vi "TDC Data Monitor def.9.vi"() -> ()   [LabVIEW 2011]
panel:
  out "Numeric 2":u32
  in  "Buffer size 2":u32=548
  out "Numeric":i32
  in  "stop 2":bool
  out "Active \nTimeout":bool
  in  "Buffer size":u32=548
  in  "Change UDP Parameters":bool
  out "Event Hex":string
  in  "see table channel  2":bool
  in  "see supertime sec":bool
  in  "see supertime  ns":bool
  in  "see channel":bool
  in  "see tot":bool
  in  "see table channel":bool
  out "error tdc not foud":bool
  out "Num Pack 2":u32=1
  out "Supertime ns":u32=1
  out "Supertime sec":u32=1
  out "error time order":bool
  out "error channel":bool
  out "Num Pack":u32=1
  out "Veces canal":u32[](array[numeric])
  out "Table":string[][](table)
  out "num canal":i32=548
  out "Canal TDC":u32[](array[numeric])
  in  "desviacion tipica ancho":dbl
  in  "suma desviacon":dbl
  out "media pulso":dbl
  in  "suma ancho pulso":u32=1
  out "iteracion":i32
  in  "stop":bool
  out "error timestamp":bool
  out "TOT":dynamicdata(graph) caption="Histogram"
  out "CHANNEL":dynamicdata(graph) caption="Histogram"
  out "ToT":u32=1
  out "Arrival Time":u32=1
  out "Channel TDC":u32=1
  out "bufferfull":timestamp
  out "UDP INDEX":dynamicdata(graph) caption="Histogram"
  out "EVENT/TS":dynamicdata(graph) caption="Histogram"
  out "indice":u32=1
  out "Supertime sec":dynamicdata(graph)
  out "supertime ns":dynamicdata(graph)
  out "current_HRV":u32=1
  out "current_fifo_afull":u32=1
  out "FIFO_FULL":bool[](array[boolean])
  out "HRV":bool[](array[boolean])
  out "Size Packet Bytes":i32
  out "Data Received":string
  out "Timeout UDP READ  ms":i32
  out "max bytes/read":i32=548
  in  "index":u32=1
  in  "Port":u16=61557
  out "Receive Buffer Size":u32
  out "Num Event":u32=1
  out "START TIME":timestamp
  out "hold_fifo_afull":u32=1
  out "hold_HRV":u32=1
  in  "event/ts":u32=1
  in  "pak_loss":u32=1 caption="packet losses"
  in  "TS_Ch_1":u32=1
  in  "TS_Ch 2":u32=1
  in  "TS_Ch 3":u32=1
  in  "TS_Ch 4":u32=1
  in  "TS_Ch 5":u32=1
  in  "TS_Ch 6":u32=1
  in  "TS_Ch 7":u32=1
  in  "TS_Ch 8":u32=1
  in  "TS_Ch 9":u32=1
  in  "TS_Ch 10":u32=1
  in  "TS_Ch_0":u32=1
  in  "TS_Ch_13":u32=1
  in  "TS_Ch 12":u32=1
  in  "TS_Ch_14":u32=1
  in  "TS_Ch_11":u32=1
  in  "TS_Ch_15":u32=1
  in  "TS_Ch_16":u32=1
  in  "TS_Ch_18":u32=1
  in  "TS_Ch 19":u32=1
  in  "TS_Ch_20":u32=1
  in  "TS_Ch_17":u32=1
  in  "TS_Ch_21":u32=1
  in  "TS_Ch_22":u32=1
  in  "TS_Ch_24":u32=1
  in  "TS_Ch 25":u32=1
  in  "TS_Ch_26":u32=1
  in  "TS_Ch_23":u32=1
  in  "TS_Ch_27":u32=1
  in  "TS_Ch_28":u32=1
  in  "TS_Ch_29":u32=1
  in  "TS_Ch_30":u32=1
  # "TDC DATA MONITOR"
  # "UDP TRANSFER CONDITIONS"
  # "PACKET INFORMATION"
  # "EVENT INFORMATION"
  # "See table of channel events"
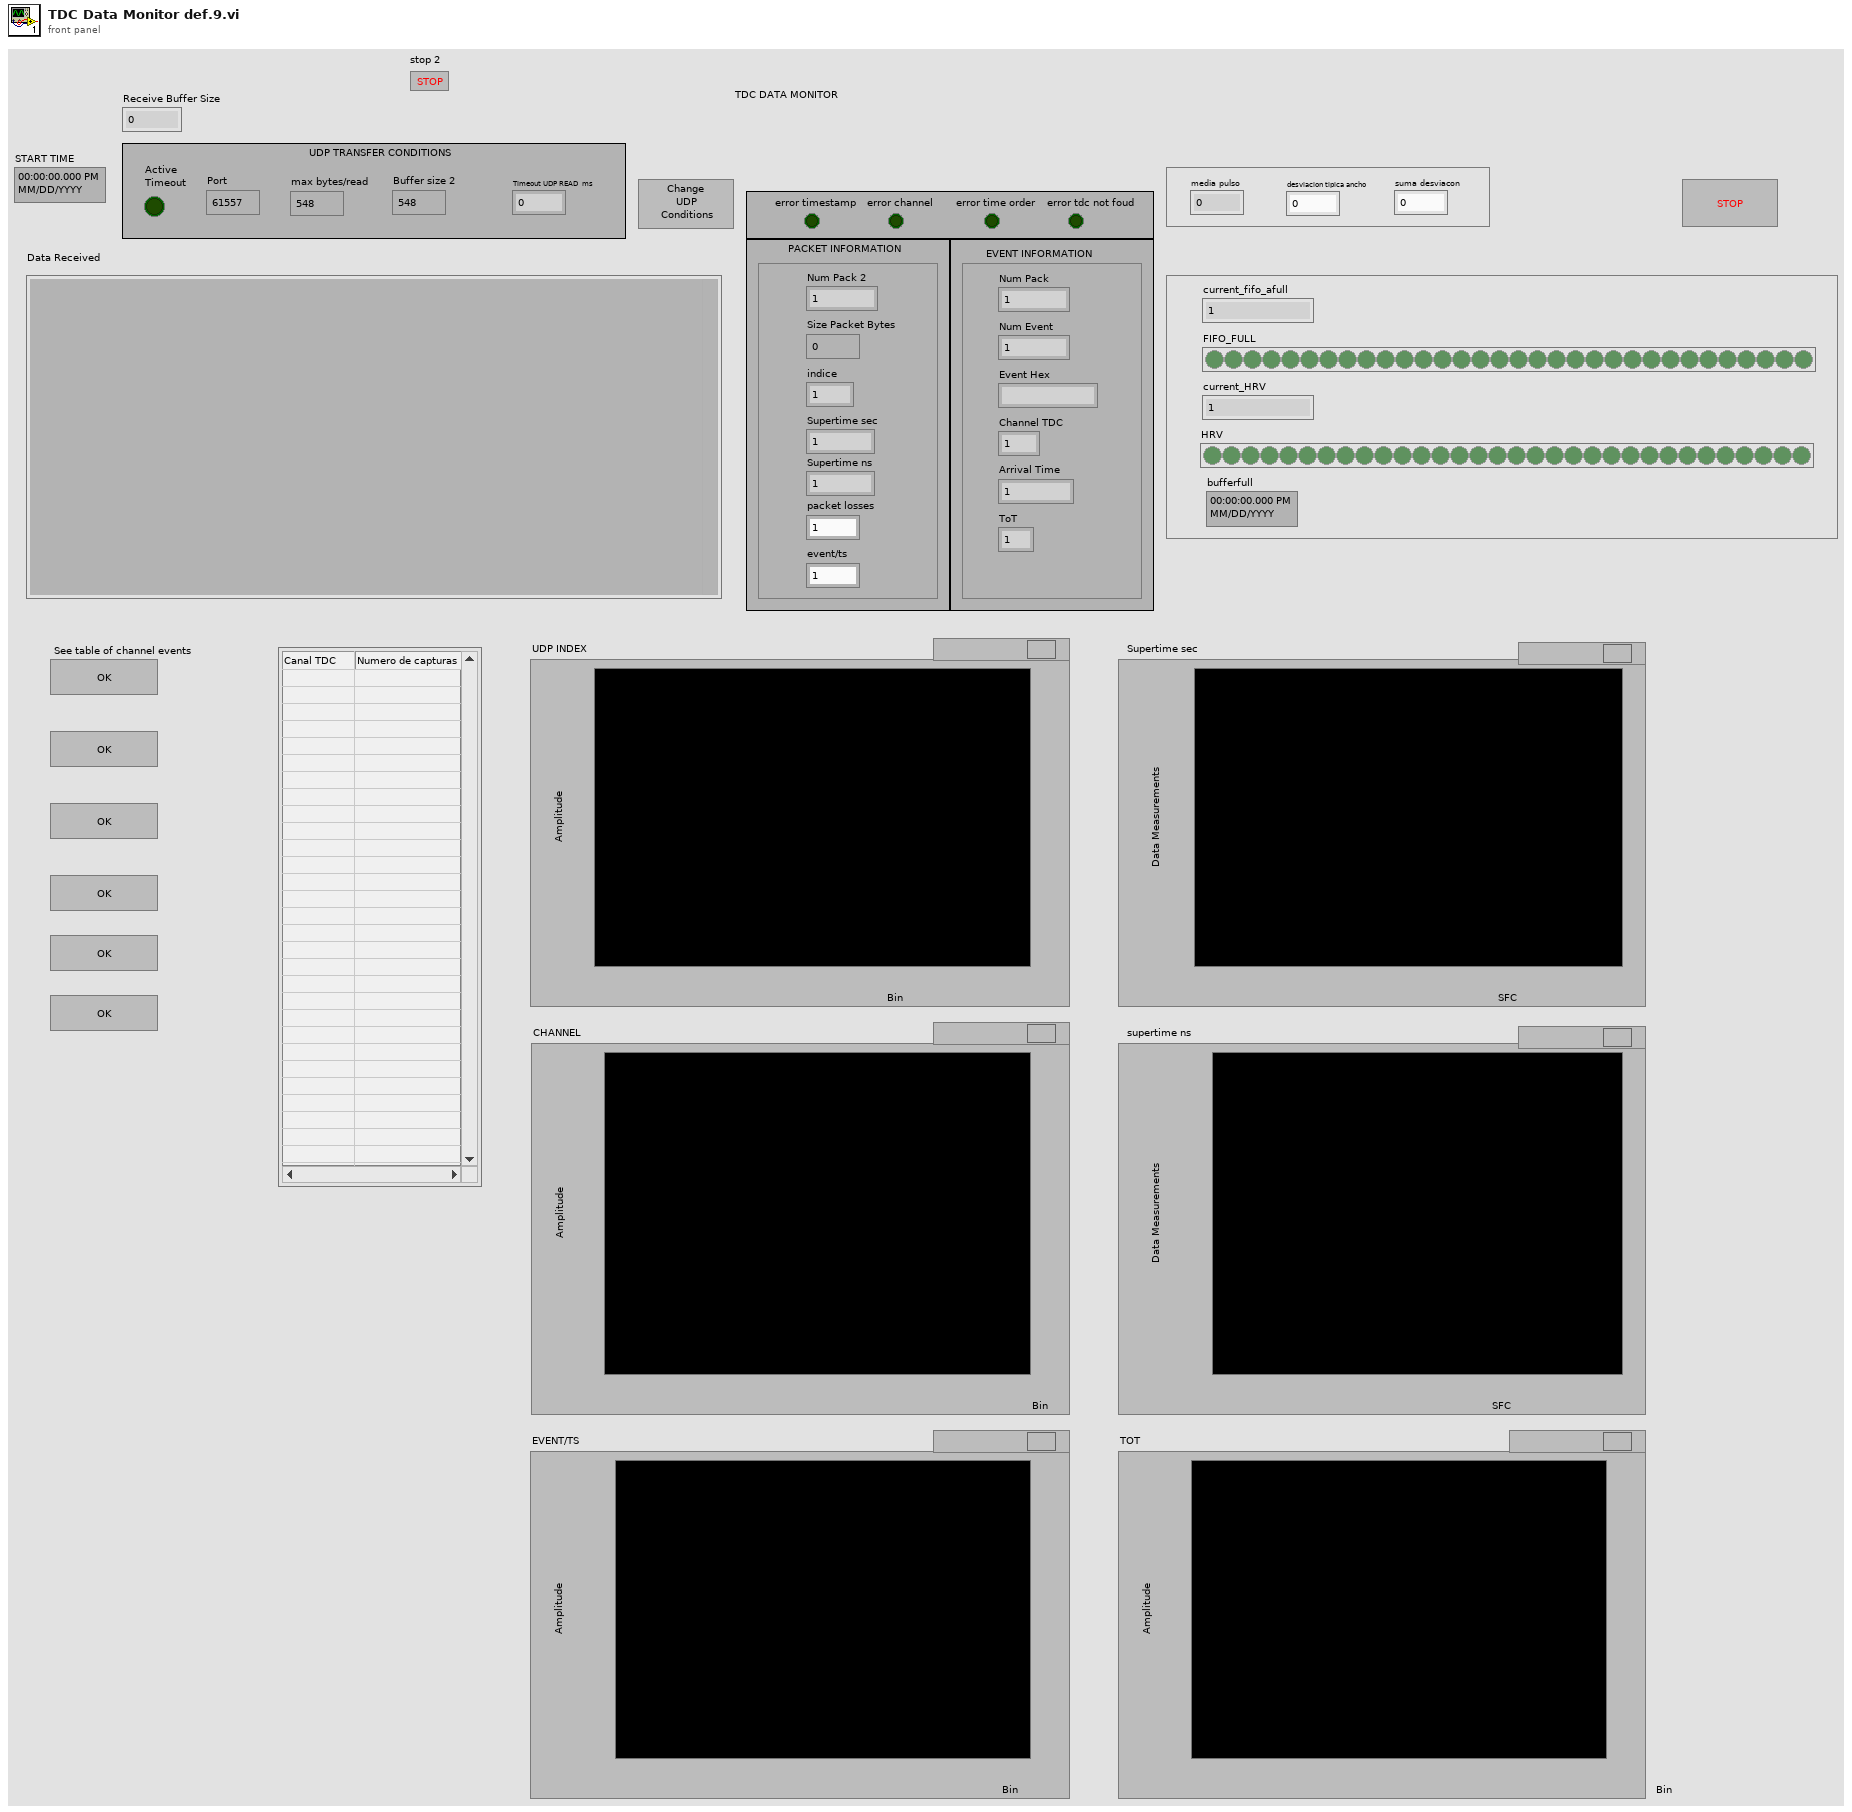
[diagram p1: front panel]
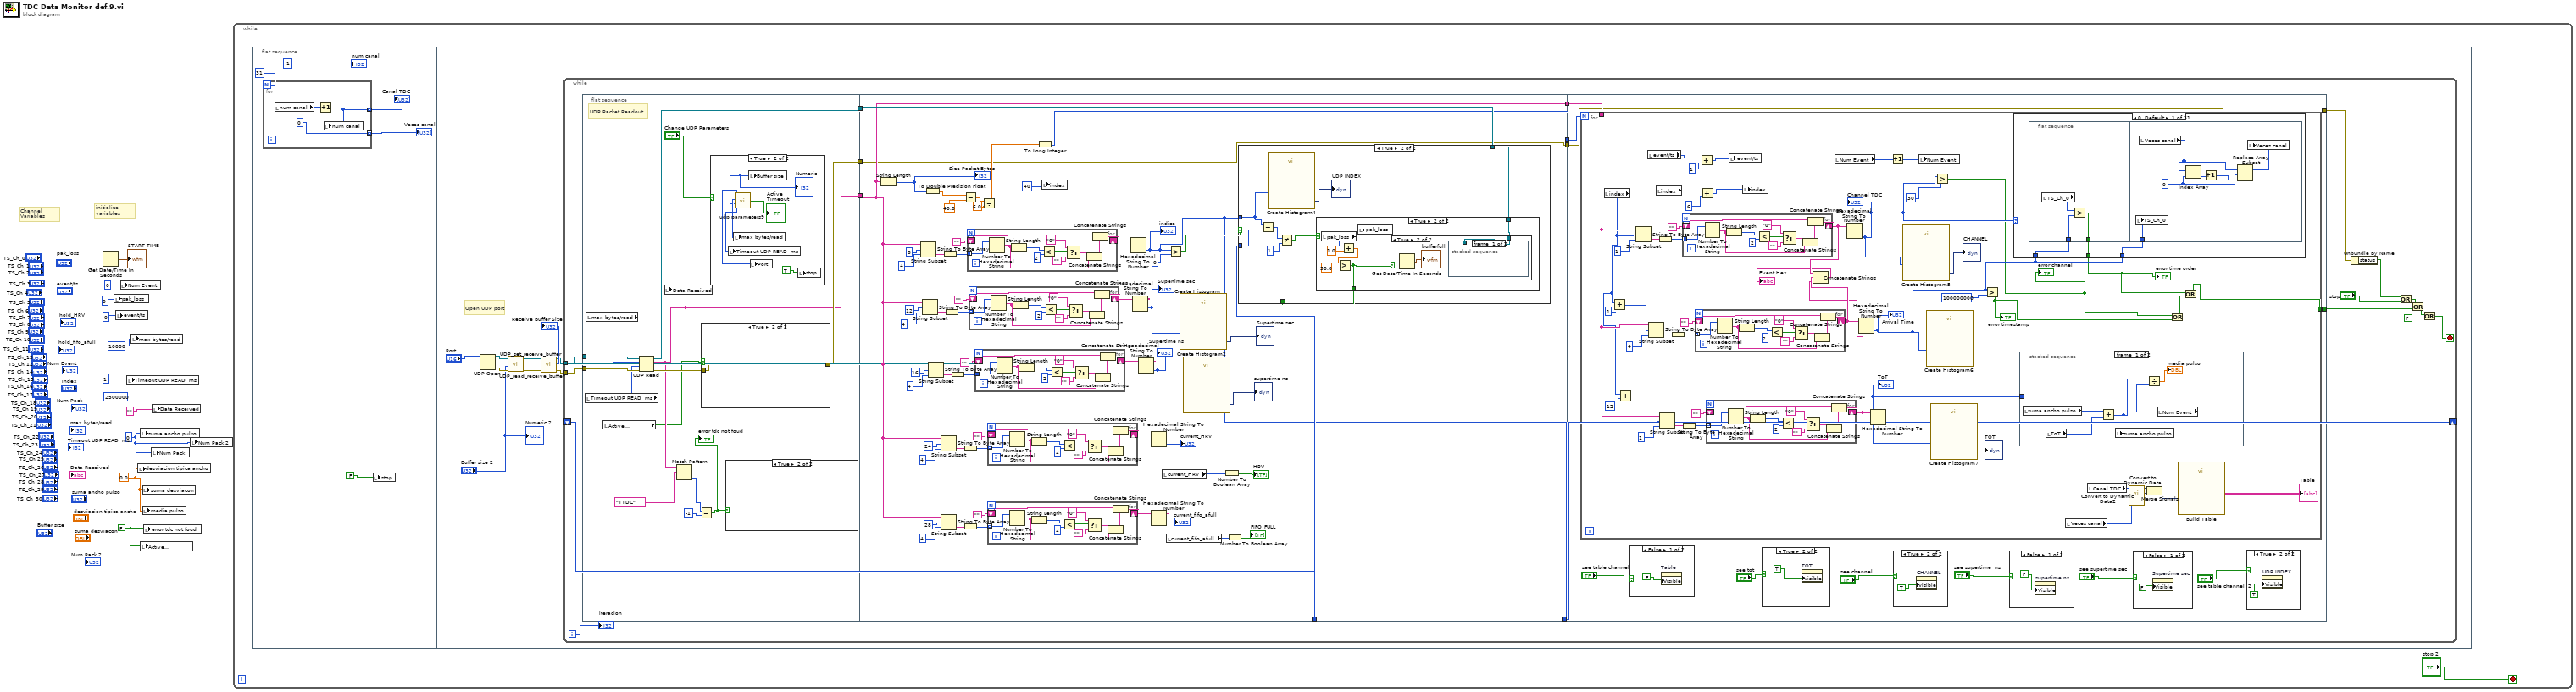
[diagram p0: block diagram]
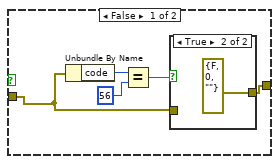
[diagram p2: hidden frame]
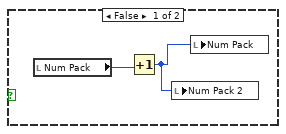
[diagram p5: hidden frame]
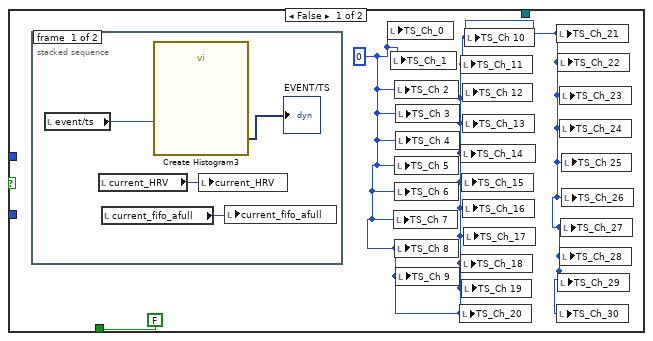
[diagram p6: hidden frame]
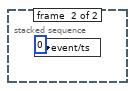
[diagram p7: hidden frame]
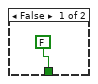
[diagram p8: hidden frame]
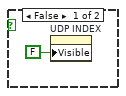
[diagram p11: hidden frame]
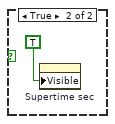
[diagram p12: hidden frame]
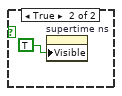
[diagram p13: hidden frame]
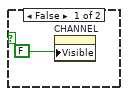
[diagram p14: hidden frame]
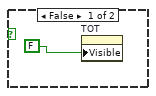
[diagram p15: hidden frame]
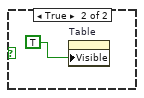
[diagram p16: hidden frame]
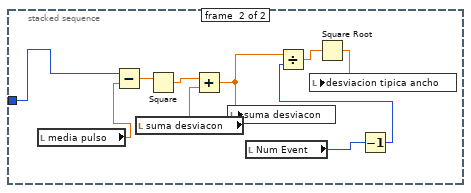
[diagram p17: hidden frame]
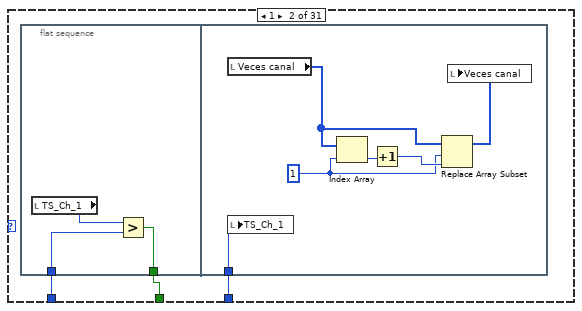
[diagram p18: hidden frame]
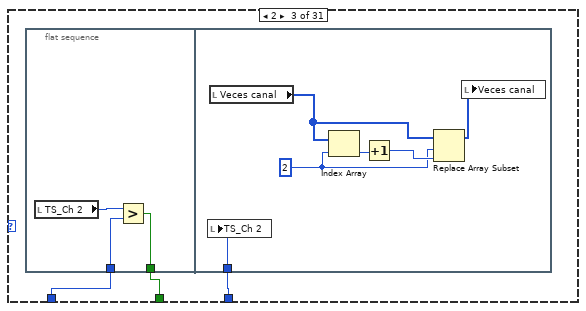
[diagram p19: hidden frame]
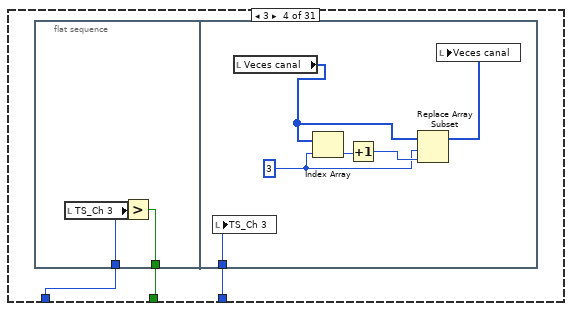
[diagram p20: hidden frame]
diagram:
  w1 = FALSE
  w3 = 0.0
  w2 = u32 0 ("event/ts")
  (unwired) u32 2500000 ("Receive Buffer Size")
  # "initialize variables"
  # "Channel Variables"
  n1 = Get Date/Time In Seconds() -> (seconds since 1Jan1904=→"START TIME":timestamp)
  n2 = local write "pak_loss"(u32 0 ("pak_loss")) -> ()
  n3 = local write "event/ts"(u32 0 ("event/ts")) -> ()
  n4 = local write "Num Event"(u32 0 ("contador eventos")) -> ()
  n5 = local write "Timeout UDP READ  ms"(1 ("event/ts")) -> ()
  n6 = local write "max bytes/read"(10000) -> ()
  n7 = local write "desviacion tipica ancho"(w3) -> ()
  n8 = local write "suma ancho pulso"(w2) -> ()
  n9 = local write "Active \nTimeout"(w1) -> ()
  n10 = local write "suma desviacon"(w3) -> ()
  n11 = local write "media pulso"(w3) -> ()
  n12 = local write "error tdc not foud"(w1) -> ()
  n13 = local write "Num Pack"(w2) -> ()
  n14 = local write "Data Received"("") -> ()
  n15 = local write "Num Pack 2"(w2) -> ()
  n16 = while {
    stop <- "stop 2" stop-if-true
    n17 = flat-sequence {
      frame #0 {
        n18 = for {
          N: 31 ("contador eventos") -> [_]
          tunnel: [w18] -> w15 mode=indexing
          tunnel: [u32 0 ("contador eventos")] -> w16 mode=indexing
          n19 = local read "num canal"() -> (w19:i32)
          n20 = Increment(x=w19) -> (x+1=w18:i32)
          n21 = local write "num canal"(w18) -> ()
        }
        "Canal TDC" <- w15
        "Veces canal" <- w16
        n22 = local write "stop"(FALSE) -> ()
        "num canal" <- -1 ("contador eventos")
      }
      frame #1 {
        # "Open UDP port"
        n23 = UDP Open(11:"Port") -> (port=w25:refnum<k16>, 0:w26:errorcluster)  [unwired: 1 in, 4 out]
        n24 = call "UDP_set_receive_buffer.vi"("error in (no error)"=w26, "Receive Buffer Size"="Buffer size 2", "connection ID"=w25) -> ("error out"=w28:errorcluster, "connection ID out"=w27:refnum<k16>)  [unwired: 6 in]
        n25 = call "UDP_read_receive_buffer.vi"("error in (no error)"=w28, "connection ID"=w27) -> ("error out"=w22:errorcluster, "Receive Buffer Size"=→"Receive Buffer Size":u32, "connection ID out"=w23:refnum<k16>)  [unwired: 5 in]
        n26 = while {
          tunnel: w23 -> [w47]
          tunnel: w22 -> [w46]
          shift-right: [w29] -> _
          shift-left: _ -> [w30]
          i -> [w31]
          stop <- w35 stop-if-true
          n27 = flat-sequence {
            tunnel: w47 -> [w61]
            tunnel: w46 -> [w60]
            tunnel: [w56] -> w45
            tunnel: [w54] -> w44
            tunnel: [w55] -> w43
            tunnel: w45 -> [w82]
            tunnel: w44 -> [w83]
            tunnel: w43 -> [w87]
            tunnel: [w84] -> w42
            tunnel: [w83] -> w41
            tunnel: [w82] -> w34
            tunnel: w30 -> [w81]
            tunnel: [w80] -> w29
            tunnel: w42 -> [w221]
            tunnel: w41 -> [w220]
            tunnel: [w219] -> w37
            tunnel: [w218] -> w33
            tunnel: w34 -> [w218]
            frame #0 {
              # "UDP Packet Readout"
              n28 = local read "Timeout UDP READ  ms"() -> (w58:i32)
              n29 = local read "max bytes/read"() -> (w59:i32)
              n30 = local read "Active \nTimeout"() -> (w48:bool)
              n31 = UDP Read(connection ID=w61, max size (548)=w59, timeout ms (25000)=w58, 8:w60) -> (data out=w54:string, error out=w57:errorcluster, 3:w55:refnum<k16>)  [unwired: 2 out]
              n32 = local write "Data Received"(w54) -> ()
              n33 = Match Pattern(string=w54, regular expression="TTDC") -> (offset past match=w50:i32)  [unwired: 1 in, 3 out]
              n34 = Equal?(x=w50, y=-1) -> (x = y?=w49:bool)
              "error tdc not foud" <- w49
              n35 = case shown="True" w48 {
                tunnel: w57 -> [w63 w69]
                tunnel: [w62 w69] -> w56
                frame False {
                  n36 = Unbundle By Name(w63) -> ("code"=w64:i32)
                  n37 = Equal?(x=w64, y=56) -> (x = y?=w66:bool)
                  n38 = case shown="True" w66 {
                    tunnel: w63 -> [w67 _]
                    tunnel: [w67 errorcluster {"status"=FALSE, "code"=0, "source"=""} ("error out")] -> w62
                    frame False {
                    }
                    frame True {
                    }
                  }
                }
                frame True {
                }
              }
              n39 = case shown="True" "Change UDP Parameters" {
                frame False {
                }
                frame True {
                  n40 = call "udp parameters9.vi"() -> ("Active Timeout UDP Read 2"=→"Active \nTimeout":bool, "Timeout UDP Read ms 2"=w75:i32, "Receive Buffer Size 2"=w70:u32, "Max Bytes/Read  2"=w74:i32, "Port 2"=w72:i32)  [unwired: 2 in]
                  "Numeric" <- w70
                  n41 = local write "Timeout UDP READ  ms"(w75) -> ()
                  n42 = local write "max bytes/read"(w74) -> ()
                  n43 = local write "Buffer size"(w70) -> ()
                  n44 = local write "Port"(w72) -> ()
                  n45 = local write "stop"(TRUE) -> ()
                }
              }
              n46 = case shown="True" w49 {
                frame False {
                  n47 = local read "Num Pack"() -> (w76:u32)
                  n48 = Increment(x=w76) -> (x+1=w77:u32)
                  n49 = local write "Num Pack 2"(w77) -> ()
                  n50 = local write "Num Pack"(w77) -> ()
                }
                frame True {
                }
              }
            }
            frame #1 {
              n51 = String Length(string=w83) -> (length=w99:i32)
              "Size Packet Bytes" <- w99
              n52 = String Subset(string=w83, offset (0)=8, length (rest)=4) -> (substring=w129:string)
              n53 = String Subset(string=w83, offset (0)=12, length (rest)=4) -> (substring=w123:string)
              n54 = To Double Precision Float(number=w99) -> (double precision float=w98:dbl)
              n55 = String Subset(string=w83, offset (0)=16, length (rest)=4) -> (substring=w117:string)
              n56 = String Subset(string=w83, offset (0)=24, length (rest)=4) -> (substring=w111:string)
              n57 = String Subset(string=w83, offset (0)=28, length (rest)=4) -> (substring=w105:string)
              n58 = String To Byte Array(string=w129) -> (unsigned byte array=w127:u8[])
              n59 = String To Byte Array(string=w123) -> (unsigned byte array=w121:u8[])
              n60 = String To Byte Array(string=w117) -> (unsigned byte array=w115:u8[])
              n61 = String To Byte Array(string=w111) -> (unsigned byte array=w109:u8[])
              n62 = String To Byte Array(string=w105) -> (unsigned byte array=w103:u8[])
              n63 = Subtract(x=w98, y=40.0) -> (x-y=w102:dbl)
              n64 = for {
                tunnel: w127 -> [w201] mode=indexing
                shift-right: [w202] -> w131
                shift-left: "" -> [w203]
                n65 = Number To Hexadecimal String(2:w201) -> (0:w205:string)  [unwired: 1 in]
                n66 = String Length(string=w205) -> (length=w211:i32)
                n67 = Less?(x=w211, y=2) -> (x < y?=w208:bool)
                n68 = Select(t="0", s=w208, f="") -> (s? t:f=w206:string)
                n69 = Concatenate Strings(w206, w205) -> (w204:string)
                n70 = Concatenate Strings(w203, w204) -> (w202:string)
              }
              n71 = for {
                tunnel: w121 -> [w190] mode=indexing
                shift-right: [w191] -> w125
                shift-left: "" -> [w192]
                n72 = Number To Hexadecimal String(2:w190) -> (0:w194:string)  [unwired: 1 in]
                n73 = String Length(string=w194) -> (length=w200:i32)
                n74 = Less?(x=w200, y=2) -> (x < y?=w197:bool)
                n75 = Select(t="0", s=w197, f="") -> (s? t:f=w195:string)
                n76 = Concatenate Strings(w195, w194) -> (w193:string)
                n77 = Concatenate Strings(w192, w193) -> (w191:string)
              }
              n78 = for {
                tunnel: w115 -> [w179] mode=indexing
                shift-right: [w180] -> w119
                shift-left: "" -> [w181]
                n79 = Number To Hexadecimal String(2:w179) -> (0:w183:string)  [unwired: 1 in]
                n80 = String Length(string=w183) -> (length=w189:i32)
                n81 = Less?(x=w189, y=2) -> (x < y?=w186:bool)
                n82 = Select(t="0", s=w186, f="") -> (s? t:f=w184:string)
                n83 = Concatenate Strings(w184, w183) -> (w182:string)
                n84 = Concatenate Strings(w181, w182) -> (w180:string)
              }
              n85 = Divide(x=w102, y=6.0) -> (x/y=w85:dbl)
              n86 = for {
                tunnel: w109 -> [w168] mode=indexing
                shift-right: [w169] -> w113
                shift-left: "" -> [w170]
                n87 = Number To Hexadecimal String(2:w168) -> (0:w172:string)  [unwired: 1 in]
                n88 = String Length(string=w172) -> (length=w178:i32)
                n89 = Less?(x=w178, y=2) -> (x < y?=w175:bool)
                n90 = Select(t="0", s=w175, f="") -> (s? t:f=w173:string)
                n91 = Concatenate Strings(w173, w172) -> (w171:string)
                n92 = Concatenate Strings(w170, w171) -> (w169:string)
              }
              n93 = for {
                tunnel: w103 -> [w157] mode=indexing
                shift-right: [w158] -> w107
                shift-left: "" -> [w159]
                n94 = Number To Hexadecimal String(2:w157) -> (0:w161:string)  [unwired: 1 in]
                n95 = String Length(string=w161) -> (length=w167:i32)
                n96 = Less?(x=w167, y=2) -> (x < y?=w164:bool)
                n97 = Select(t="0", s=w164, f="") -> (s? t:f=w162:string)
                n98 = Concatenate Strings(w162, w161) -> (w160:string)
                n99 = Concatenate Strings(w159, w160) -> (w158:string)
              }
              n100 = To Long Integer(number=w85) -> (32bit integer=w84:i32)
              n101 = local write "index"(u32 40 ("index")) -> ()
              n102 = Hexadecimal String To Number(string=w131) -> (number=w80:u32)  [unwired: 2 in, 1 out]
              "indice" <- w80
              n103 = Hexadecimal String To Number(string=w125) -> (number=w79:u32)  [unwired: 2 in, 1 out]
              "Supertime sec" <- w79
              n104 = Hexadecimal String To Number(string=w119) -> (number=w78:u32)  [unwired: 2 in, 1 out]
              "Supertime ns" <- w78
              n105 = Hexadecimal String To Number(string=w113) -> (number=→"current_HRV":u32)  [unwired: 2 in, 1 out]
              n106 = Hexadecimal String To Number(string=w107) -> (number=→"current_fifo_afull":u32)  [unwired: 2 in, 1 out]
              n107 = local read "current_HRV"() -> (w90:u32)
              n108 = local read "current_fifo_afull"() -> (w89:u32)
              n109 = Greater?(x=w80, y=u32 0 ("index")) -> (0:w86:bool)
              n110 = call "Create Histogram"("Signal"=w79) -> ("Histogram"=→"Supertime sec":dynamicdata)  [unwired: 9 in, 1 out]
              n111 = call "Create Histogram2"("Signal"=w78) -> ("Histogram"=→"supertime ns":dynamicdata)  [unwired: 9 in, 1 out]
              n112 = Number To Boolean Array(number=w90) -> (Boolean array=→"HRV":bool[])
              n113 = Number To Boolean Array(number=w89) -> (Boolean array=→"FIFO_FULL":bool[])
              n114 = case shown="True" w86 {
                tunnel: w80 -> [_ w141]
                tunnel: w81 -> [_ w147]
                tunnel: [FALSE w144] -> _
                tunnel: w87 -> [_ w143]
                frame False {
                  w133 = u32 0 ("TS_Ch 10")
                  n115 = stacked-sequence {
                    frame #0 {
                      n116 = local read "event/ts"() -> (w137:u32)
                      n117 = local read "current_HRV"() -> (w136:u32)
                      n118 = local read "current_fifo_afull"() -> (w135:u32)
                      n119 = call "Create Histogram3"("Signal"=w137) -> ("Histogram"=→"EVENT/TS":dynamicdata)  [unwired: 9 in, 1 out]
                      n120 = local write "current_HRV"(w136) -> ()
                      n121 = local write "current_fifo_afull"(w135) -> ()
                    }
                    frame #1 {
                      n122 = local write "event/ts"(u32 0 ("event/ts")) -> ()
                    }
                  }
                  n123 = local write "TS_Ch_0"(w133) -> ()
                  n124 = local write "TS_Ch_1"(w133) -> ()
                  n125 = local write "TS_Ch 7"(w133) -> ()
                  n126 = local write "TS_Ch 2"(w133) -> ()
                  n127 = local write "TS_Ch 5"(w133) -> ()
                  n128 = local write "TS_Ch 6"(w133) -> ()
                  n129 = local write "TS_Ch 8"(w133) -> ()
                  n130 = local write "TS_Ch 3"(w133) -> ()
                  n131 = local write "TS_Ch 4"(w133) -> ()
                  n132 = local write "TS_Ch 9"(w133) -> ()
                  n133 = local write "TS_Ch_20"(w133) -> ()
                  n134 = local write "TS_Ch_11"(w133) -> ()
                  n135 = local write "TS_Ch_14"(w133) -> ()
                  n136 = local write "TS_Ch_18"(w133) -> ()
                  n137 = local write "TS_Ch_15"(w133) -> ()
                  n138 = local write "TS_Ch 19"(w133) -> ()
                  n139 = local write "TS_Ch 12"(w133) -> ()
                  n140 = local write "TS_Ch_13"(w133) -> ()
                  n141 = local write "TS_Ch_16"(w133) -> ()
                  n142 = local write "TS_Ch_17"(w133) -> ()
                  n143 = local write "TS_Ch 10"(w133) -> ()
                  n144 = local write "TS_Ch_21"(w133) -> ()
                  n145 = local write "TS_Ch_30"(w133) -> ()
                  n146 = local write "TS_Ch_22"(w133) -> ()
                  n147 = local write "TS_Ch_29"(w133) -> ()
                  n148 = local write "TS_Ch_23"(w133) -> ()
                  n149 = local write "TS_Ch_24"(w133) -> ()
                  n150 = local write "TS_Ch_28"(w133) -> ()
                  n151 = local write "TS_Ch_27"(w133) -> ()
                  n152 = local write "TS_Ch 25"(w133) -> ()
                  n153 = local write "TS_Ch_26"(w133) -> ()
                }
                frame True {
                  n154 = Subtract(x=w141, y=w147) -> (x-y=w146:u32)
                  n155 = call "Create Histogram4"("Signal"=w141) -> ("Histogram"=→"UDP INDEX":dynamicdata)  [unwired: 9 in, 1 out]
                  n156 = Not Equal?(x=w146, y=u32 1) -> (x != y?=w140:bool)
                  n157 = case shown="True" w140 {
                    tunnel: [FALSE w150] -> w144
                    tunnel: w143 -> [_ w149]
                    frame False {
                    }
                    frame True {
                      n158 = local read "pak_loss"() -> (w154:u32)
                      n159 = Add(x=w154, y=1.0) -> (x+y=w151:dbl)
                      n160 = Greater?(x=w151, y=50.0) -> (0:w150:bool)
                      n161 = local write "pak_loss"(w151) -> ()
                      n162 = case shown="True" w150 {
                        tunnel: w149 -> [_ w155]
                        frame False {
                        }
                        frame True {
                          n163 = Get Date/Time In Seconds() -> (seconds since 1Jan1904=→"bufferfull":timestamp)
                          n164 = stacked-sequence {
                            tunnel: w155 -> [_ _]
                            frame #0 {
                            }
                            frame #1 {
                            }
                          }
                        }
                      }
                    }
                  }
                }
              }
            }
            frame #2 {
              n165 = for {
                N: w221 -> [_]
                tunnel: w220 -> [w269]
                tunnel: [w255] -> w219
                n166 = local read "index"() -> (w249:u32)
                n167 = Add(x=w249, y=u32 1) -> (x+y=w252:u32)
                n168 = Add(x=w249, y=12 ("offset (0)")) -> (x+y=w251:u32)
                n169 = String Subset(string=w269, offset (0)=w249, length (rest)=1) -> (substring=w280:string)
                n170 = local read "event/ts"() -> (w268:u32)
                n171 = String Subset(string=w269, offset (0)=w252, length (rest)=4) -> (substring=w276:string)
                n172 = local read "index"() -> (w254:u32)
                n173 = String To Byte Array(string=w280) -> (unsigned byte array=w278:u8[])
                n174 = String Subset(string=w269, offset (0)=w251, length (rest)=1) -> (substring=w272:string)
                n175 = String To Byte Array(string=w276) -> (unsigned byte array=w274:u8[])
                n176 = String To Byte Array(string=w272) -> (unsigned byte array=w270:u8[])
                n177 = for {
                  tunnel: w278 -> [w691] mode=indexing
                  shift-right: [w692] -> w237
                  shift-left: "" -> [w693]
                  n178 = Number To Hexadecimal String(2:w691) -> (0:w695:string)  [unwired: 1 in]
                  n179 = String Length(string=w695) -> (length=w701:i32)
                  n180 = Less?(x=w701, y=2) -> (x < y?=w698:bool)
                  n181 = Select(t="0", s=w698, f="") -> (s? t:f=w696:string)
                  n182 = Concatenate Strings(w696, w695) -> (w694:string)
                  n183 = Concatenate Strings(w693, w694) -> (w692:string)
                }
                n184 = for {
                  tunnel: w274 -> [w680] mode=indexing
                  shift-right: [w681] -> w236
                  shift-left: "" -> [w682]
                  n185 = Number To Hexadecimal String(2:w680) -> (0:w684:string)  [unwired: 1 in]
                  n186 = String Length(string=w684) -> (length=w690:i32)
                  n187 = Less?(x=w690, y=2) -> (x < y?=w687:bool)
                  n188 = Select(t="0", s=w687, f="") -> (s? t:f=w685:string)
                  n189 = Concatenate Strings(w685, w684) -> (w683:string)
                  n190 = Concatenate Strings(w682, w683) -> (w681:string)
                }
                n191 = Add(x=w268, y=u32 1) -> (x+y=w267:u32)
                n192 = Add(x=w254, y=u32 6) -> (x+y=w264:u32)
                n193 = for {
                  tunnel: w270 -> [w669] mode=indexing
                  shift-right: [w670] -> w235
                  shift-left: "" -> [w671]
                  n194 = Number To Hexadecimal String(2:w669) -> (0:w673:string)  [unwired: 1 in]
                  n195 = String Length(string=w673) -> (length=w679:i32)
                  n196 = Less?(x=w679, y=2) -> (x < y?=w676:bool)
                  n197 = Select(t="0", s=w676, f="") -> (s? t:f=w674:string)
                  n198 = Concatenate Strings(w674, w673) -> (w672:string)
                  n199 = Concatenate Strings(w671, w672) -> (w670:string)
                }
                n200 = local write "event/ts"(w267) -> ()
                n201 = local write "index"(w264) -> ()
                n202 = Concatenate Strings(w237, w236, w235) -> (→"Event Hex":string)
                n203 = local read "Num Event"() -> (w260:u32)
                n204 = Hexadecimal String To Number(string=w237) -> (number=w243:u32)  [unwired: 2 in, 1 out]
                "Channel TDC" <- w243
                n205 = Hexadecimal String To Number(string=w236) -> (number=w256:u32)  [unwired: 2 in, 1 out]
                "Arrival Time" <- w256
                n206 = Hexadecimal String To Number(string=w235) -> (number=w247:u32)  [unwired: 2 in, 1 out]
                "ToT" <- w247
                n207 = Increment(x=w260) -> (x+1=w259:u32)
                n208 = call "Create Histogram5"("Signal"=w243) -> ("Histogram"=→"CHANNEL":dynamicdata)  [unwired: 9 in, 1 out]
                n209 = local write "Num Event"(w259) -> ()
                n210 = call "Create Histogram6"("Signal"=w256) -> ()  [unwired: 9 in, 2 out]
                n211 = call "Create Histogram7"("Signal"=w247) -> ("Histogram"=→"TOT":dynamicdata)  [unwired: 9 in, 1 out]
                n212 = Greater?(x=w243, y=u32 30) -> (0:w239:bool)
                "error channel" <- w239
                n213 = Greater?(x=w256, y=u32 100000000 ("x")) -> (0:w258:bool)
                "error timestamp" <- w258
                n214 = case shown="0, Default" w243 {
                  tunnel: w256 -> [w298 w311 w322 w334 w346 w358 w370 w382 w394 w406 w418 w430 w442 w454 w466 w478 w490 w502 w514 w526 w538 w550 w562 w574 w586 w598 w610 w622 w634 w646 w659]
                  tunnel: w256 -> [w299 w310 w323 w335 w347 w359 w371 w383 w395 w407 w419 w431 w443 w455 w467 w479 w491 w503 w515 w527 w539 w551 w563 w575 w587 w599 w611 w623 w635 w647 w658]
                  tunnel: [w297 w309 w321 w333 w345 w357 w369 w381 w393 w405 w417 w429 w441 w453 w465 w477 w489 w501 w513 w525 w537 w549 w561 w573 w585 w597 w609 w621 w633 w645 w657] -> w238
                  frame 0, Default {
                    n215 = flat-sequence {
                      tunnel: w299 -> [w301]
                      tunnel: [w300] -> w297
                      tunnel: w298 -> [w308]
                      frame #0 {
                        n216 = local read "TS_Ch_0"() -> (w302:u32)
                        n217 = Greater?(x=w302, y=w301) -> (0:w300:bool)
                      }
                      frame #1 {
                        w305 = 0 ("contador eventos")
                        n218 = local write "TS_Ch_0"(w308) -> ()
                        n219 = local read "Veces canal"() -> (w304:u32[])
                        n220 = Index Array(array=w304, index=w305) -> (element=w306:u32)
                        n221 = Increment(x=w306) -> (x+1=w307:u32)
                        n222 = Replace Array Subset(array=w304, new element=w307, index=w305) -> (w303:u32[])
                        n223 = local write "Veces canal"(w303) -> ()
                      }
                    }
                  }
                  frame 1 {
                    n224 = flat-sequence {
                      tunnel: w310 -> [w314]
                      tunnel: [w312] -> w309
                      tunnel: w311 -> [w320]
                      frame #0 {
                        n225 = local read "TS_Ch_1"() -> (w313:u32)
                        n226 = Greater?(x=w313, y=w314) -> (0:w312:bool)
                      }
                      frame #1 {
                        w317 = 1 ("contador eventos")
                        n227 = local read "Veces canal"() -> (w316:u32[])
                        n228 = local write "TS_Ch_1"(w320) -> ()
                        n229 = Index Array(array=w316, index=w317) -> (element=w318:u32)
                        n230 = Increment(x=w318) -> (x+1=w319:u32)
                        n231 = Replace Array Subset(array=w316, new element=w319, index=w317) -> (w315:u32[])
                        n232 = local write "Veces canal"(w315) -> ()
                      }
                    }
                  }
                  frame 2 {
                    n233 = flat-sequence {
                      tunnel: w323 -> [w325]
                      tunnel: [w324] -> w321
                      tunnel: w322 -> [w332]
                      frame #0 {
                        n234 = local read "TS_Ch 2"() -> (w326:u32)
                        n235 = Greater?(x=w326, y=w325) -> (0:w324:bool)
                      }
                      frame #1 {
                        w327 = 2 ("contador eventos")
                        n236 = local write "TS_Ch 2"(w332) -> ()
                        n237 = local read "Veces canal"() -> (w330:u32[])
                        n238 = Index Array(array=w330, index=w327) -> (element=w328:u32)
                        n239 = Increment(x=w328) -> (x+1=w329:u32)
                        n240 = Replace Array Subset(array=w330, new element=w329, index=w327) -> (w331:u32[])
                        n241 = local write "Veces canal"(w331) -> ()
                      }
                    }
                  }
                  frame 3 {
                    n242 = flat-sequence {
                      tunnel: w335 -> [w337]
                      tunnel: [w336] -> w333
                      tunnel: w334 -> [w344]
                      frame #0 {
                        n243 = local read "TS_Ch 3"() -> (w338:u32)
                        n244 = Greater?(x=w338, y=w337) -> (0:w336:bool)
                      }
                      frame #1 {
                        w341 = 3 ("contador eventos")
                        n245 = local write "TS_Ch 3"(w344) -> ()
                        n246 = local read "Veces canal"() -> (w340:u32[])
                        n247 = Index Array(array=w340, index=w341) -> (element=w342:u32)
                        n248 = Increment(x=w342) -> (x+1=w343:u32)
                        n249 = Replace Array Subset(array=w340, new element=w343, index=w341) -> (w339:u32[])
                        n250 = local write "Veces canal"(w339) -> ()
                      }
                    }
                  }
                  frame 4 {
                    n251 = flat-sequence {
                      tunnel: w347 -> [w349]
                      tunnel: [w348] -> w345
                      tunnel: w346 -> [w356]
                      frame #0 {
                        n252 = local read "TS_Ch 4"() -> (w350:u32)
                        n253 = Greater?(x=w350, y=w349) -> (0:w348:bool)
                      }
                      frame #1 {
                        w353 = 4 ("contador eventos")
                        n254 = local write "TS_Ch 4"(w356) -> ()
                        n255 = local read "Veces canal"() -> (w352:u32[])
                        n256 = Index Array(array=w352, index=w353) -> (element=w354:u32)
                        n257 = Increment(x=w354) -> (x+1=w355:u32)
                        n258 = Replace Array Subset(array=w352, new element=w355, index=w353) -> (w351:u32[])
                        n259 = local write "Veces canal"(w351) -> ()
                      }
                    }
                  }
                  frame 5 {
                    n260 = flat-sequence {
                      tunnel: w359 -> [w361]
                      tunnel: [w360] -> w357
                      tunnel: w358 -> [w368]
                      frame #0 {
                        n261 = local read "TS_Ch 5"() -> (w362:u32)
                        n262 = Greater?(x=w362, y=w361) -> (0:w360:bool)
                      }
                      frame #1 {
                        w365 = 5 ("contador eventos")
                        n263 = local write "TS_Ch 5"(w368) -> ()
                        n264 = local read "Veces canal"() -> (w364:u32[])
                        n265 = Index Array(array=w364, index=w365) -> (element=w366:u32)
                        n266 = Increment(x=w366) -> (x+1=w367:u32)
                        n267 = Replace Array Subset(array=w364, new element=w367, index=w365) -> (w363:u32[])
                        n268 = local write "Veces canal"(w363) -> ()
                      }
                    }
                  }
                  frame 6 {
                    n269 = flat-sequence {
                      tunnel: w371 -> [w373]
                      tunnel: [w372] -> w369
                      tunnel: w370 -> [w380]
                      frame #0 {
                        n270 = local read "TS_Ch 6"() -> (w374:u32)
                        n271 = Greater?(x=w374, y=w373) -> (0:w372:bool)
                      }
                      frame #1 {
                        w377 = 6 ("contador eventos")
                        n272 = local write "TS_Ch 6"(w380) -> ()
                        n273 = local read "Veces canal"() -> (w376:u32[])
                        n274 = Index Array(array=w376, index=w377) -> (element=w378:u32)
                        n275 = Increment(x=w378) -> (x+1=w379:u32)
                        n276 = Replace Array Subset(array=w376, new element=w379, index=w377) -> (w375:u32[])
                        n277 = local write "Veces canal"(w375) -> ()
                      }
                    }
                  }
                  frame 7 {
                    n278 = flat-sequence {
                      tunnel: w383 -> [w385]
                      tunnel: [w384] -> w381
                      tunnel: w382 -> [w392]
                      frame #0 {
                        n279 = local read "TS_Ch 7"() -> (w386:u32)
                        n280 = Greater?(x=w386, y=w385) -> (0:w384:bool)
                      }
                      frame #1 {
                        w389 = 7 ("contador eventos")
                        n281 = local write "TS_Ch 7"(w392) -> ()
                        n282 = local read "Veces canal"() -> (w388:u32[])
                        n283 = Index Array(array=w388, index=w389) -> (element=w390:u32)
                        n284 = Increment(x=w390) -> (x+1=w391:u32)
                        n285 = Replace Array Subset(array=w388, new element=w391, index=w389) -> (w387:u32[])
                        n286 = local write "Veces canal"(w387) -> ()
                      }
                    }
                  }
                  frame 8 {
                    n287 = flat-sequence {
                      tunnel: w395 -> [w397]
                      tunnel: [w396] -> w393
                      tunnel: w394 -> [w404]
                      frame #0 {
                        n288 = local read "TS_Ch 8"() -> (w398:u32)
                        n289 = Greater?(x=w398, y=w397) -> (0:w396:bool)
                      }
                      frame #1 {
                        w401 = 8 ("contador eventos")
                        n290 = local write "TS_Ch 8"(w404) -> ()
                        n291 = local read "Veces canal"() -> (w400:u32[])
                        n292 = Index Array(array=w400, index=w401) -> (element=w402:u32)
                        n293 = Increment(x=w402) -> (x+1=w403:u32)
                        n294 = Replace Array Subset(array=w400, new element=w403, index=w401) -> (w399:u32[])
                        n295 = local write "Veces canal"(w399) -> ()
                      }
                    }
                  }
                  frame 9 {
                    n296 = flat-sequence {
                      tunnel: w407 -> [w409]
                      tunnel: [w408] -> w405
                      tunnel: w406 -> [w416]
                      frame #0 {
                        n297 = local read "TS_Ch 9"() -> (w410:u32)
                        n298 = Greater?(x=w410, y=w409) -> (0:w408:bool)
                      }
                      frame #1 {
                        w413 = 9 ("contador eventos")
                        n299 = local write "TS_Ch 9"(w416) -> ()
                        n300 = local read "Veces canal"() -> (w412:u32[])
                        n301 = Index Array(array=w412, index=w413) -> (element=w414:u32)
                        n302 = Increment(x=w414) -> (x+1=w415:u32)
                        n303 = Replace Array Subset(array=w412, new element=w415, index=w413) -> (w411:u32[])
                        n304 = local write "Veces canal"(w411) -> ()
                      }
                    }
                  }
                  frame 10 {
                    n305 = flat-sequence {
                      tunnel: w419 -> [w421]
                      tunnel: [w420] -> w417
                      tunnel: w418 -> [w428]
                      frame #0 {
                        n306 = local read "TS_Ch 10"() -> (w422:u32)
                        n307 = Greater?(x=w422, y=w421) -> (0:w420:bool)
                      }
                      frame #1 {
                        w425 = 10 ("contador eventos")
                        n308 = local write "TS_Ch 10"(w428) -> ()
                        n309 = local read "Veces canal"() -> (w424:u32[])
                        n310 = Index Array(array=w424, index=w425) -> (element=w426:u32)
                        n311 = Increment(x=w426) -> (x+1=w427:u32)
                        n312 = Replace Array Subset(array=w424, new element=w427, index=w425) -> (w423:u32[])
                        n313 = local write "Veces canal"(w423) -> ()
                      }
                    }
                  }
                  frame 11 {
                    n314 = flat-sequence {
                      tunnel: w431 -> [w433]
                      tunnel: [w432] -> w429
                      tunnel: w430 -> [w440]
                      frame #0 {
                        n315 = local read "TS_Ch_11"() -> (w434:u32)
                        n316 = Greater?(x=w434, y=w433) -> (0:w432:bool)
                      }
                      frame #1 {
                        w437 = 11 ("contador eventos")
                        n317 = local write "TS_Ch_11"(w440) -> ()
                        n318 = local read "Veces canal"() -> (w435:u32[])
                        n319 = Index Array(array=w435, index=w437) -> (element=w438:u32)
                        n320 = Increment(x=w438) -> (x+1=w439:u32)
                        n321 = Replace Array Subset(array=w435, new element=w439, index=w437) -> (w436:u32[])
                        n322 = local write "Veces canal"(w436) -> ()
                      }
                    }
                  }
                  frame 12 {
                    n323 = flat-sequence {
                      tunnel: w443 -> [w445]
                      tunnel: [w444] -> w441
                      tunnel: w442 -> [w452]
                      frame #0 {
                        n324 = local read "TS_Ch 12"() -> (w446:u32)
                        n325 = Greater?(x=w446, y=w445) -> (0:w444:bool)
                      }
                      frame #1 {
                        w449 = 12 ("contador eventos")
                        n326 = local read "Veces canal"() -> (w447:u32[])
                        n327 = local write "TS_Ch 12"(w452) -> ()
                        n328 = Index Array(array=w447, index=w449) -> (element=w450:u32)
                        n329 = Increment(x=w450) -> (x+1=w451:u32)
                        n330 = Replace Array Subset(array=w447, new element=w451, index=w449) -> (w448:u32[])
                        n331 = local write "Veces canal"(w448) -> ()
                      }
                    }
                  }
                  frame 13 {
                    n332 = flat-sequence {
                      tunnel: w455 -> [w457]
                      tunnel: [w456] -> w453
                      tunnel: w454 -> [w464]
                      frame #0 {
                        n333 = local read "TS_Ch_13"() -> (w458:u32)
                        n334 = Greater?(x=w458, y=w457) -> (0:w456:bool)
                      }
                      frame #1 {
                        w461 = 13 ("contador eventos")
                        n335 = local read "Veces canal"() -> (w459:u32[])
                        n336 = local write "TS_Ch_13"(w464) -> ()
                        n337 = Index Array(array=w459, index=w461) -> (element=w462:u32)
                        n338 = Increment(x=w462) -> (x+1=w463:u32)
                        n339 = Replace Array Subset(array=w459, new element=w463, index=w461) -> (w460:u32[])
                        n340 = local write "Veces canal"(w460) -> ()
                      }
                    }
                  }
                  frame 14 {
                    n341 = flat-sequence {
                      tunnel: w467 -> [w469]
                      tunnel: [w468] -> w465
                      tunnel: w466 -> [w476]
                      frame #0 {
                        n342 = local read "TS_Ch_14"() -> (w470:u32)
                        n343 = Greater?(x=w470, y=w469) -> (0:w468:bool)
                      }
                      frame #1 {
                        w473 = 14 ("contador eventos")
                        n344 = local write "TS_Ch_14"(w476) -> ()
                        n345 = local read "Veces canal"() -> (w471:u32[])
                        n346 = Index Array(array=w471, index=w473) -> (element=w474:u32)
                        n347 = Increment(x=w474) -> (x+1=w475:u32)
                        n348 = Replace Array Subset(array=w471, new element=w475, index=w473) -> (w472:u32[])
                        n349 = local write "Veces canal"(w472) -> ()
                      }
                    }
                  }
                  frame 15 {
                    n350 = flat-sequence {
                      tunnel: w479 -> [w481]
                      tunnel: [w480] -> w477
                      tunnel: w478 -> [w488]
                      frame #0 {
                        n351 = local read "TS_Ch_15"() -> (w482:u32)
                        n352 = Greater?(x=w482, y=w481) -> (0:w480:bool)
                      }
                      frame #1 {
                        w485 = 15 ("contador eventos")
                        n353 = local write "TS_Ch_15"(w488) -> ()
                        n354 = local read "Veces canal"() -> (w483:u32[])
                        n355 = Index Array(array=w483, index=w485) -> (element=w486:u32)
                        n356 = Increment(x=w486) -> (x+1=w487:u32)
                        n357 = Replace Array Subset(array=w483, new element=w487, index=w485) -> (w484:u32[])
                        n358 = local write "Veces canal"(w484) -> ()
                      }
                    }
                  }
                  frame 16 {
                    n359 = flat-sequence {
                      tunnel: w491 -> [w493]
                      tunnel: [w492] -> w489
                      tunnel: w490 -> [w500]
                      frame #0 {
                        n360 = local read "TS_Ch_16"() -> (w494:u32)
                        n361 = Greater?(x=w494, y=w493) -> (0:w492:bool)
                      }
                      frame #1 {
                        w497 = 16 ("contador eventos")
                        n362 = local write "TS_Ch_16"(w500) -> ()
                        n363 = local read "Veces canal"() -> (w495:u32[])
                        n364 = Index Array(array=w495, index=w497) -> (element=w498:u32)
                        n365 = Increment(x=w498) -> (x+1=w499:u32)
                        n366 = Replace Array Subset(array=w495, new element=w499, index=w497) -> (w496:u32[])
                        n367 = local write "Veces canal"(w496) -> ()
                      }
                    }
                  }
                  frame 17 {
                    n368 = flat-sequence {
                      tunnel: w503 -> [w505]
                      tunnel: [w504] -> w501
                      tunnel: w502 -> [w512]
                      frame #0 {
                        n369 = local read "TS_Ch_17"() -> (w506:u32)
                        n370 = Greater?(x=w506, y=w505) -> (0:w504:bool)
                      }
                      frame #1 {
                        w509 = 17 ("contador eventos")
                        n371 = local write "TS_Ch_17"(w512) -> ()
                        n372 = local read "Veces canal"() -> (w507:u32[])
                        n373 = Index Array(array=w507, index=w509) -> (element=w510:u32)
                        n374 = Increment(x=w510) -> (x+1=w511:u32)
                        n375 = Replace Array Subset(array=w507, new element=w511, index=w509) -> (w508:u32[])
                        n376 = local write "Veces canal"(w508) -> ()
                      }
                    }
                  }
                  frame 18 {
                    n377 = flat-sequence {
                      tunnel: w515 -> [w517]
                      tunnel: [w516] -> w513
                      tunnel: w514 -> [w524]
                      frame #0 {
                        n378 = local read "TS_Ch_18"() -> (w518:u32)
                        n379 = Greater?(x=w518, y=w517) -> (0:w516:bool)
                      }
                      frame #1 {
                        w521 = 18 ("contador eventos")
                        n380 = local write "TS_Ch_18"(w524) -> ()
                        n381 = local read "Veces canal"() -> (w519:u32[])
                        n382 = Index Array(array=w519, index=w521) -> (element=w522:u32)
                        n383 = Increment(x=w522) -> (x+1=w523:u32)
                        n384 = Replace Array Subset(array=w519, new element=w523, index=w521) -> (w520:u32[])
                        n385 = local write "Veces canal"(w520) -> ()
                      }
                    }
                  }
                  frame 19 {
                    n386 = flat-sequence {
                      tunnel: w527 -> [w529]
                      tunnel: [w528] -> w525
                      tunnel: w526 -> [w536]
                      frame #0 {
                        n387 = local read "TS_Ch 19"() -> (w530:u32)
                        n388 = Greater?(x=w530, y=w529) -> (0:w528:bool)
                      }
                      frame #1 {
                        w533 = 19 ("contador eventos")
                        n389 = local write "TS_Ch 19"(w536) -> ()
                        n390 = local read "Veces canal"() -> (w532:u32[])
                        n391 = Index Array(array=w532, index=w533) -> (element=w534:u32)
                        n392 = Increment(x=w534) -> (x+1=w535:u32)
                        n393 = Replace Array Subset(array=w532, new element=w535, index=w533) -> (w531:u32[])
                        n394 = local write "Veces canal"(w531) -> ()
                      }
                    }
                  }
                  frame 20 {
                    n395 = flat-sequence {
                      tunnel: w539 -> [w541]
                      tunnel: [w540] -> w537
                      tunnel: w538 -> [w548]
                      frame #0 {
                        n396 = local read "TS_Ch_20"() -> (w542:u32)
                        n397 = Greater?(x=w542, y=w541) -> (0:w540:bool)
                      }
                      frame #1 {
                        w545 = 20 ("contador eventos")
                        n398 = local write "TS_Ch_20"(w548) -> ()
                        n399 = local read "Veces canal"() -> (w544:u32[])
                        n400 = Index Array(array=w544, index=w545) -> (element=w546:u32)
                        n401 = Increment(x=w546) -> (x+1=w547:u32)
                        n402 = Replace Array Subset(array=w544, new element=w547, index=w545) -> (w543:u32[])
                        n403 = local write "Veces canal"(w543) -> ()
                      }
                    }
                  }
                  frame 21 {
                    n404 = flat-sequence {
                      tunnel: w551 -> [w553]
                      tunnel: [w552] -> w549
                      tunnel: w550 -> [w560]
                      frame #0 {
                        n405 = local read "TS_Ch_21"() -> (w554:u32)
                        n406 = Greater?(x=w554, y=w553) -> (0:w552:bool)
                      }
                      frame #1 {
                        w557 = 21 ("contador eventos")
                        n407 = local write "TS_Ch_21"(w560) -> ()
                        n408 = local read "Veces canal"() -> (w556:u32[])
                        n409 = Index Array(array=w556, index=w557) -> (element=w558:u32)
                        n410 = Increment(x=w558) -> (x+1=w559:u32)
                        n411 = Replace Array Subset(array=w556, new element=w559, index=w557) -> (w555:u32[])
                        n412 = local write "Veces canal"(w555) -> ()
                      }
                    }
                  }
                  frame 22 {
                    n413 = flat-sequence {
                      tunnel: w563 -> [w565]
                      tunnel: [w564] -> w561
                      tunnel: w562 -> [w572]
                      frame #0 {
                        n414 = local read "TS_Ch_22"() -> (w566:u32)
                        n415 = Greater?(x=w566, y=w565) -> (0:w564:bool)
                      }
                      frame #1 {
                        w569 = 22 ("contador eventos")
                        n416 = local read "Veces canal"() -> (w567:u32[])
                        n417 = local write "TS_Ch_22"(w572) -> ()
                        n418 = Index Array(array=w567, index=w569) -> (element=w570:u32)
                        n419 = Increment(x=w570) -> (x+1=w571:u32)
                        n420 = Replace Array Subset(array=w567, new element=w571, index=w569) -> (w568:u32[])
                        n421 = local write "Veces canal"(w568) -> ()
                      }
                    }
                  }
                  frame 23 {
                    n422 = flat-sequence {
                      tunnel: w575 -> [w577]
                      tunnel: [w576] -> w573
                      tunnel: w574 -> [w584]
                      frame #0 {
                        n423 = local read "TS_Ch_23"() -> (w578:u32)
                        n424 = Greater?(x=w578, y=w577) -> (0:w576:bool)
                      }
                      frame #1 {
                        w581 = 23 ("contador eventos")
                        n425 = local read "Veces canal"() -> (w579:u32[])
                        n426 = local write "TS_Ch_23"(w584) -> ()
                        n427 = Index Array(array=w579, index=w581) -> (element=w582:u32)
                        n428 = Increment(x=w582) -> (x+1=w583:u32)
                        n429 = Replace Array Subset(array=w579, new element=w583, index=w581) -> (w580:u32[])
                        n430 = local write "Veces canal"(w580) -> ()
                      }
                    }
                  }
                  frame 24 {
                    n431 = flat-sequence {
                      tunnel: w587 -> [w589]
                      tunnel: [w588] -> w585
                      tunnel: w586 -> [w596]
                      frame #0 {
                        n432 = local read "TS_Ch_24"() -> (w590:u32)
                        n433 = Greater?(x=w590, y=w589) -> (0:w588:bool)
                      }
                      frame #1 {
                        w593 = 24 ("contador eventos")
                        n434 = local write "TS_Ch_24"(w596) -> ()
                        n435 = local read "Veces canal"() -> (w591:u32[])
                        n436 = Index Array(array=w591, index=w593) -> (element=w594:u32)
                        n437 = Increment(x=w594) -> (x+1=w595:u32)
                        n438 = Replace Array Subset(array=w591, new element=w595, index=w593) -> (w592:u32[])
                        n439 = local write "Veces canal"(w592) -> ()
                      }
                    }
                  }
                  frame 25 {
                    n440 = flat-sequence {
                      tunnel: w599 -> [w601]
                      tunnel: [w600] -> w597
                      tunnel: w598 -> [w608]
                      frame #0 {
                        n441 = local read "TS_Ch 25"() -> (w602:u32)
                        n442 = Greater?(x=w602, y=w601) -> (0:w600:bool)
                      }
                      frame #1 {
                        w605 = 25 ("contador eventos")
                        n443 = local write "TS_Ch 25"(w608) -> ()
                        n444 = local read "Veces canal"() -> (w603:u32[])
                        n445 = Index Array(array=w603, index=w605) -> (element=w606:u32)
                        n446 = Increment(x=w606) -> (x+1=w607:u32)
                        n447 = Replace Array Subset(array=w603, new element=w607, index=w605) -> (w604:u32[])
                        n448 = local write "Veces canal"(w604) -> ()
                      }
                    }
                  }
                  frame 26 {
                    n449 = flat-sequence {
                      tunnel: w611 -> [w613]
                      tunnel: [w612] -> w609
                      tunnel: w610 -> [w620]
                      frame #0 {
                        n450 = local read "TS_Ch_26"() -> (w614:u32)
                        n451 = Greater?(x=w614, y=w613) -> (0:w612:bool)
                      }
                      frame #1 {
                        w617 = 26 ("contador eventos")
                        n452 = local write "TS_Ch_26"(w620) -> ()
                        n453 = local read "Veces canal"() -> (w615:u32[])
                        n454 = Index Array(array=w615, index=w617) -> (element=w618:u32)
                        n455 = Increment(x=w618) -> (x+1=w619:u32)
                        n456 = Replace Array Subset(array=w615, new element=w619, index=w617) -> (w616:u32[])
                        n457 = local write "Veces canal"(w616) -> ()
                      }
                    }
                  }
                  frame 27 {
                    n458 = flat-sequence {
                      tunnel: w623 -> [w625]
                      tunnel: [w624] -> w621
                      tunnel: w622 -> [w632]
                      frame #0 {
                        n459 = local read "TS_Ch_27"() -> (w626:u32)
                        n460 = Greater?(x=w626, y=w625) -> (0:w624:bool)
                      }
                      frame #1 {
                        w629 = 27 ("contador eventos")
                        n461 = local write "TS_Ch_27"(w632) -> ()
                        n462 = local read "Veces canal"() -> (w628:u32[])
                        n463 = Index Array(array=w628, index=w629) -> (element=w630:u32)
                        n464 = Increment(x=w630) -> (x+1=w631:u32)
                        n465 = Replace Array Subset(array=w628, new element=w631, index=w629) -> (w627:u32[])
                        n466 = local write "Veces canal"(w627) -> ()
                      }
                    }
                  }
                  frame 28 {
                    n467 = flat-sequence {
                      tunnel: w635 -> [w637]
                      tunnel: [w636] -> w633
                      tunnel: w634 -> [w644]
                      frame #0 {
                        n468 = local read "TS_Ch_28"() -> (w638:u32)
                        n469 = Greater?(x=w638, y=w637) -> (0:w636:bool)
                      }
                      frame #1 {
                        w641 = 28 ("contador eventos")
                        n470 = local read "Veces canal"() -> (w639:u32[])
                        n471 = local write "TS_Ch_28"(w644) -> ()
                        n472 = Index Array(array=w639, index=w641) -> (element=w642:u32)
                        n473 = Increment(x=w642) -> (x+1=w643:u32)
                        n474 = Replace Array Subset(array=w639, new element=w643, index=w641) -> (w640:u32[])
                        n475 = local write "Veces canal"(w640) -> ()
                      }
                    }
                  }
                  frame 29 {
                    n476 = flat-sequence {
                      tunnel: w647 -> [w649]
                      tunnel: [w648] -> w645
                      tunnel: w646 -> [w656]
                      frame #0 {
                        n477 = local read "TS_Ch_29"() -> (w650:u32)
                        n478 = Greater?(x=w650, y=w649) -> (0:w648:bool)
                      }
                      frame #1 {
                        w653 = 29 ("contador eventos")
                        n479 = local write "TS_Ch_29"(w656) -> ()
                        n480 = local read "Veces canal"() -> (w651:u32[])
                        n481 = Index Array(array=w651, index=w653) -> (element=w654:u32)
                        n482 = Increment(x=w654) -> (x+1=w655:u32)
                        n483 = Replace Array Subset(array=w651, new element=w655, index=w653) -> (w652:u32[])
                        n484 = local write "Veces canal"(w652) -> ()
                      }
                    }
                  }
                  frame 30 {
                    n485 = flat-sequence {
                      tunnel: [w661] -> w657
                      tunnel: w658 -> [w660]
                      tunnel: w659 -> [w668]
                      frame #0 {
                        n486 = local read "TS_Ch_30"() -> (w662:u32)
                        n487 = Greater?(x=w662, y=w660) -> (0:w661:bool)
                      }
                      frame #1 {
                        w665 = 30 ("contador eventos")
                        n488 = local read "Veces canal"() -> (w664:u32[])
                        n489 = local write "TS_Ch_30"(w668) -> ()
                        n490 = Index Array(array=w664, index=w665) -> (element=w666:u32)
                        n491 = Increment(x=w666) -> (x+1=w667:u32)
                        n492 = Replace Array Subset(array=w664, new element=w667, index=w665) -> (w663:u32[])
                        n493 = local write "Veces canal"(w663) -> ()
                      }
                    }
                  }
                }
                "error time order" <- w238
                n494 = stacked-sequence {
                  tunnel: w247 -> [_ w287]
                  frame #0 {
                    n495 = local read "suma ancho pulso"() -> (w286:u32)
                    n496 = local read "ToT"() -> (w285:u32)
                    n497 = Add(x=w286, y=w285) -> (x+y=w284:u32)
                    n498 = local write "suma ancho pulso"(w284) -> ()
                    n499 = local read "Num Event"() -> (w283:u32)
                    n500 = Divide(x=w284, y=w283) -> (x/y=→"media pulso":dbl)
                  }
                  frame #1 {
                    n501 = local read "media pulso"() -> (w296:dbl)
                    n502 = Subtract(x=w287, y=w296) -> (x-y=w295:dbl)
                    n503 = local read "suma desviacon"() -> (w293:dbl)
                    n504 = Square(x=w295) -> (x^2=w294:dbl)
                    n505 = Add(x=w294, y=w293) -> (x+y=w292:dbl)
                    n506 = local write "suma desviacon"(w292) -> ()
                    n507 = local read "Num Event"() -> (w291:u32)
                    n508 = Decrement(x=w291) -> (x-1=w290:u32)
                    n509 = Divide(x=w292, y=w290) -> (x/y=w289:dbl)
                    n510 = Square Root(x=w289) -> (sqrt(x)=w288:dbl)
                    n511 = local write "desviacion tipica ancho"(w288) -> ()
                  }
                }
                n512 = local read "Veces canal"() -> (w241:u32[])
                n513 = local read "Canal TDC"() -> (w246:u32[])
                n514 = call "Convert to Dynamic Data"("Array"=w246) -> ("Dynamic Data Type"=w245:dynamicdata)  [unwired: 3 in]
                n515 = call "Convert to Dynamic Data2"("Array"=w241) -> ("Dynamic Data Type"=w240:dynamicdata)  [unwired: 3 in]
                n516 = Merge Signals(w245, w240) -> (w244:dynamicdata)
                n517 = Or(x=w239, y=w258) -> (x .or. y?=w257:bool)
                n518 = call "Build Table"("Signals"=w244) -> ("Table"=→"Table":string[][])  [unwired: 9 in, 1 out]
                n519 = Or(x=w238, y=w257) -> (x .or. y?=w255:bool)
              }
              n520 = case shown="False" "see table channel" {
                frame False {
                  n521 = property on="Table" class="Tbl (strict)"("Visible"=FALSE) -> ()  [unwired: 2 in, 2 out]
                }
                frame True {
                  n522 = property on="Table" class="Tbl (strict)"("Visible"=TRUE) -> ()  [unwired: 2 in, 2 out]
                }
              }
              n523 = case shown="True" "see tot" {
                frame False {
                  n524 = property on="TOT" class="WFGraph (strict)"("Visible"=FALSE) -> ()  [unwired: 2 in, 2 out]
                }
                frame True {
                  n525 = property on="TOT" class="WFGraph (strict)"("Visible"=TRUE) -> ()  [unwired: 2 in, 2 out]
                }
              }
              n526 = case shown="True" "see channel" {
                frame False {
                  n527 = property on="CHANNEL" class="WFGraph (strict)"("Visible"=FALSE) -> ()  [unwired: 2 in, 2 out]
                }
                frame True {
                  n528 = property on="CHANNEL" class="WFGraph (strict)"("Visible"=TRUE) -> ()  [unwired: 2 in, 2 out]
                }
              }
              n529 = case shown="False" "see supertime  ns" {
                frame False {
                  n530 = property on="supertime ns" class="WFGraph (strict)"("Visible"=FALSE) -> ()  [unwired: 2 in, 2 out]
                }
                frame True {
                  n531 = property on="supertime ns" class="WFGraph (strict)"("Visible"=TRUE) -> ()  [unwired: 2 in, 2 out]
                }
              }
              n532 = case shown="False" "see supertime sec" {
                frame False {
                  n533 = property on="Supertime sec" class="WFGraph (strict)"("Visible"=FALSE) -> ()  [unwired: 2 in, 2 out]
                }
                frame True {
                  n534 = property on="Supertime sec" class="WFGraph (strict)"("Visible"=TRUE) -> ()  [unwired: 2 in, 2 out]
                }
              }
              n535 = case shown="True" "see table channel  2" {
                frame False {
                  n536 = property on="UDP INDEX" class="WFGraph (strict)"("Visible"=FALSE) -> ()  [unwired: 2 in, 2 out]
                }
                frame True {
                  n537 = property on="UDP INDEX" class="WFGraph (strict)"("Visible"=TRUE) -> ()  [unwired: 2 in, 2 out]
                }
              }
            }
          }
          n538 = Unbundle By Name(w33) -> ("status"=w32:bool)
          n539 = Or(x=w32, y="stop") -> (x .or. y?=w38:bool)
          n540 = Or(x=w38, y=w37) -> (x .or. y?=w39:bool)
          n541 = Or(x=w39, y=FALSE) -> (x .or. y?=w35:bool)
          "iteracion" <- w31
        }
        "Numeric 2" <- "Buffer size 2"
      }
    }
  }
